vi "get pelletron voltage from c and v.vi"(9 "Mass":ext, 10 "Velocity":sgl, 11 "Charge":sgl) -> (3 "High Voltage (MV)":sgl)   [LabVIEW 2012]
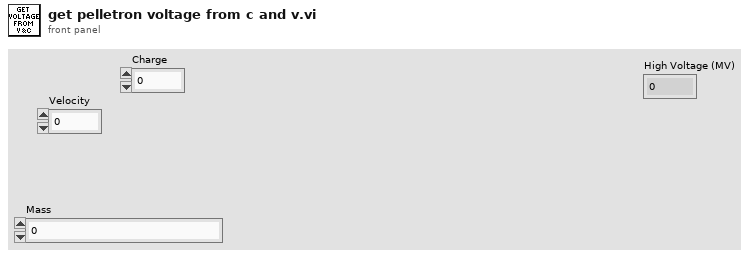
[diagram p1: front panel]
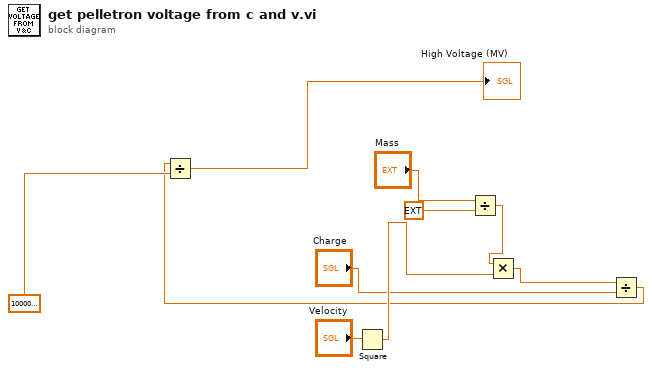
[diagram p0: block diagram]
diagram:
  n1 = Square(x="Velocity") -> (x^2=w4:sgl)
  n2 = Divide(x="Mass", y=ext 2.0) -> (x/y=w5:ext)
  n3 = Multiply(x=w5, y=w4) -> (x*y=w3:ext)
  n4 = Divide(x=w3, y="Charge") -> (x/y=w1:ext)
  n5 = Divide(x=w1, y=sgl 1000000.0) -> (x/y=→"High Voltage (MV)":ext)
